vi "InterpretLocation.vi"(10 "y":i32, 11 "x":i32) -> (3 "Numeric":i32)   [LabVIEW 2018]
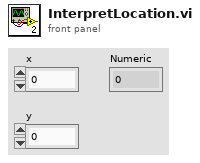
[diagram p1: front panel]
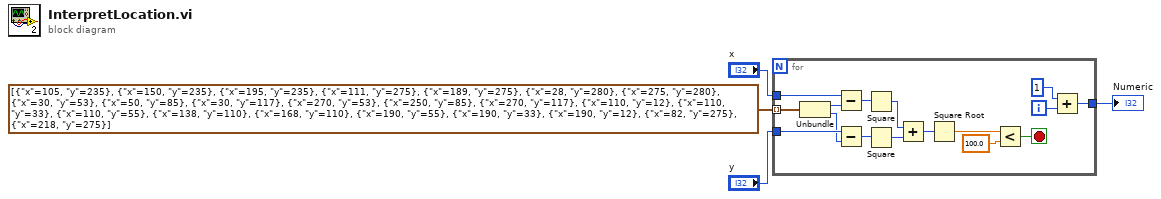
[diagram p0: block diagram]
diagram:
  n1 = for {
    tunnel: "x" -> [w16]
    tunnel: "y" -> [w15]
    tunnel: [w18] -> w4
    tunnel: cluster{"x":i32, "y":i32}[] [{"x"=105, "y"=235}, {"x"=150, "y"=235}, {"x"=195, "y"=235}, {"x"=111, "y"=275}, {"x"=189, "y"=275}, {"x"=28, "y"=280}, {"x"=275, "y"=280}, {"x"=30, "y"=53}, {"x"=50, "y"=85}, {"x"=30, "y"=117}, {"x"=270, "y"=53}, {"x"=250, "y"=85}, {"x"=270, "y"=117}, {"x"=110, "y"=12}, {"x"=110, "y"=33}, {"x"=110, "y"=55}, {"x"=138, "y"=110}, {"x"=168, "y"=110}, {"x"=190, "y"=55}, {"x"=190, "y"=33}, {"x"=190, "y"=12}, {"x"=82, "y"=275}, {"x"=218, "y"=275}] -> [w17] mode=indexing
    i -> [w20]
    stop <- w5 stop-if-true
    n2 = Unbundle(w17) -> ("x"=w14:i32, "y"=w13:i32)
    n3 = Subtract(x=w16, y=w14) -> (x-y=w12:i32)
    n4 = Subtract(x=w15, y=w13) -> (x-y=w11:i32)
    n5 = Square(x=w12) -> (x^2=w9:i32)
    n6 = Square(x=w11) -> (x^2=w10:i32)
    n7 = Add(x=w9, y=w10) -> (x+y=w8:i32)
    n8 = Square Root(x=w8) -> (sqrt(x)=w7:dbl)
    n9 = Less?(x=w7, y=100.0) -> (x < y?=w5:bool)
    n10 = Add(x=1, y=w20) -> (x+y=w18:i32)
  }
  "Numeric" <- w4
